vi "Register for Broadcasting Events Recursively.vi"(8 "error in (no error)":errorcluster, 11 "Application in":refnum<class "Application.lvclass">) -> (0 "error out":errorcluster, 2 "Event Registration Refnum":refnum<event-registration>, 3 "Application out":refnum<class "Application.lvclass">)   [LabVIEW 2020, in "Application.lvclass"]
doc: "Register for the broad cast events for the application and nested processes."
uses:
  Application.lvclass
  Process/Protected/Broadcasting/Broadcast Message Cluster.ctl
  Process/Process.lvclass
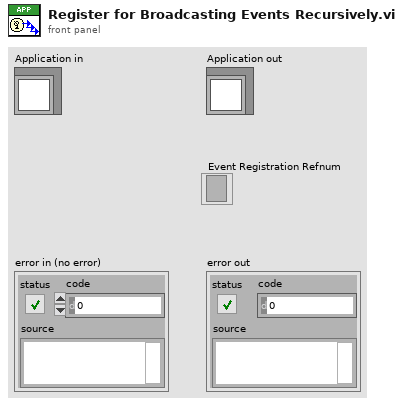
[diagram p1: front panel]
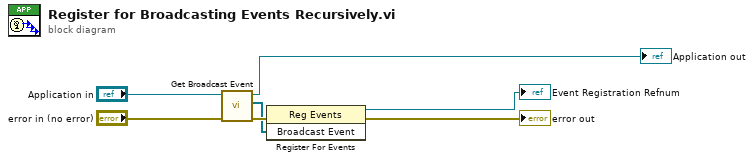
[diagram p0: block diagram]
diagram:
  n1 = call-dynamic "Get Broadcast Event.vi"("error in (no error)"="error in (no error)", "Application in"="Application in") -> ("error out"=w6:errorcluster, "Broadcast Event"=w5:refnum<user-event>[], "Application out"=→"Application out":refnum<class "Application.lvclass">)  [unwired: 7 in]
  n2 = register-events(error in=w6, w5) -> (reference out=→"Event Registration Refnum":refnum<event-registration>, error out=→"error out":errorcluster)  [unwired: 1 in]
